vi "Robot Global Data.vi"() -> ()   [LabVIEW 2016]
doc: "This global VI can contain as many global variables as you need. Place a control on the panel, give it a good name. To read or write to it from a VI, drag the icon to the diagram of that VI. You can also drag from the project. Click on the node to change which global you access. You shouldn't have multiple locations writing to a global or it will cause a race-condition."
uses:
  <vilib>/Rock Robotics/WPI/Camera/WPI_CameraImageSize.ctl
  <vilib>/Rock Robotics/WPI/DriverStation/WPI_DriverStationRobotMode2.ctl
panel:
  in  "Stop Command?":bool
  in  "Motor Power":dbl
  in  "Motor Control":T1(ring)
  in  "Jog Mode?":bool
  in  "Shooter RPM":dbl
  in  "NavX Data":T2
  in  "Collision Impact":dbl
  in  "Ultrasonic Distance":dbl
  in  "Robot Mode":T3
  in  "image size":T4=enum."320x240"
  in  "Enable Vision":bool
  # "Whoops, you found it"
  # "Shady, aftermath\nThere she goes shaking that ass on the floor\nBumpin' and grindin' that pole\nThe way she's grindin' that pole, I think I'm losing control\n\nGet buzzed, get drunk, get crunked, get fucked up\nHit the strip club don't forget once get your dick rubbed\nGet fucked, get sucked, get wasted, shit faceted\nPasted, blasted, puke drink up, get a new drink\nHit the bathroom sink, throw up\nWipe your shoe clean, got a routine\nKnowin' still got a few chunks on your shoestring\nKnowin' I was dehydrated till the beat vibrated\nI was revibed as soon as this bitch is gyrated\nAnd hips and licked them lips and that was it\nI had to get Nate Dogg and his sing some shit\n\nTwo to the one from the one to the three\nI like good pussy and I like good trees\nSmoke so much weed you wouldn't believe\nAnd I get more ass than a toilet seat\nThree to the one from the one to the three\nI met a bad bitch last night in the D\nLet me tell you how I made her leave with me\nConversation and Hennessey\nI've been to the muthafuckin' mountain top\nHeard muthafuckers talk, seen and dropped\nIf I ain't got a weapon I'm a pick up a rock\nAnd when I bust yo ass I'm a continue to rock\nGetcha ass of the wall with your two left feet\nIt's real easy just follow the beat\nDon't let that fine girl pass you by\nLook real close cause strobe lights lie\n\nWe 'bout to have a party (turn the music up)\nLet's get it started (Go head shake your butt)\nI'm lookin' for a girl with a body and a sexy strut\nWanna get it poppin' baby step right up\nSome girls they act retarded\nSome girls are bout it bout it\nI'm lookin' for a girl that will do whatever the fuck\nI say everyday she be givin' it up\n\nShake that ass for me, shake that ass for me\nCome on girl, shake that ass for me, shake that ass for me\nOh girl, shake that ass for me, shake that ass for me\nCome on girl, shake that ass for me, shake that ass for me\n\nI'm a menace, a dentist, an oral hygienist\nOpen your mouth for about four or five minutes\nTake a little bit of this fluoride with it\nSwish but don't spit it, swallow and I'll finish\nYeah me and Nate d-o double g\nLooking for a couple bitches with some double d's\nPop a little champagne and a couple E's\nSlip it in her bubbuly, we finna finna have a party\n\nWe 'bout to have a party (turn the music up)\nLet's get it started (Go head shake your butt)\nI'm lookin' for a girl I can fuck in my hummer truck\nApple Bottom jeans and a big ol' slut\nSome girls they act retarded\nSome girls are bout it 'bout it\nI want a bitch that sit at the crib with no panties on\nKnows that she can say no but she won't say no\nNow look at this lady all in front of me, sexy as can be\nTonight I want a slut, will you be mine?\nI heard you was freaky from a friend of mine\n\nNow I hope you don't get mad at me\nBut I told Nate you was a freak\nHe said he wants a slut, hope you don't mind\nI told him that you like it from behind\n\nNow, shake that ass for me, shake that ass for me\nC'mon girl, shake that ass for me, shake that ass for me\nOh girl, shake that ass for me, shake that ass for me\nC'mon girl, shake that ass for me, shake that ass for me\nWe bout' to have a party (turn the music up)\nLet's get it started (go ahead shake that butt)\nI'm lookin' for a girl with a body and a sexy strut\nWanna get it poppin' baby step right up\nSome girls they act retarded\nSome girls are bout it bout it\nI'm lookin' for a girl that will do whatever the fuck\nI say everyday she be givin' it up\n\nThere she goes, shaking that ass on the floor\nBumpin' and grindin' that pole\nThe way she's grindin' that pole\nI think I'm losing control\n\nGod, come one,\nI ain't leavin' without you bitch\nYou're coming home with me\nAnd my boy,\nAnd his boy,\nAnd his boy,\nAnd his girl"
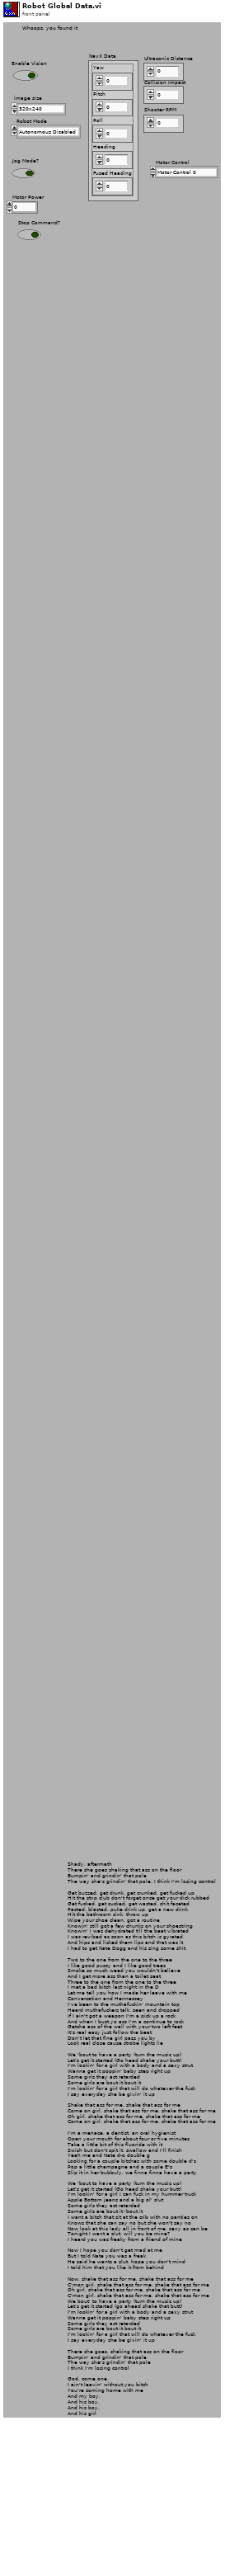
[diagram p1: front panel]
types:
  T1 = enum16{"Motor Control 0", "Motor Control 1", "Motor Control 2", "Motor Control 3", "Motor Control 4", "Motor Control 5", "Motor Control 6", "Motor Control 7"}
  T2 = cluster{"Yaw":dbl, "Pitch":dbl, "Roll":dbl, "Heading":dbl, "Fused Heading":dbl}
  T3 = typedef "WPI_DriverStationRobotMode2.ctl" = enum16{"Autonomous Disabled", "Autonomous Enabled", "Teleop Disabled", "Teleop Enabled", "Disconnected", "Finish", "Test Disabled", "Test Enabled", "Emergency Stopped"}
  T4 = typedef "WPI_CameraImageSize.ctl" = enum16{"640x480", "320x240", "160x120", "Custom"}
diagram:
